vi "Open Dev Ex.vi"(7 "FuncNo":u8, 9 "DevNo":u8, 10 "busNo":u8, 11 "devId":i32) -> (2 "function return":i32, 3 "devId out":i32)   [LabVIEW 2013, in "CHR34XXX.lvlib"]
doc: "DLL BOOL __stdcall CHR34XXX_OpenDev(IN int devId); DLL BOOL __stdcall CHR34XXX_OpenDevEx(OUT int *devId,IN BYTE busNo,IN BYTE DevNo,IN BYTE FuncNo);"
uses:
  CHR34XXX.lvlib
  CHR34XXX.dll
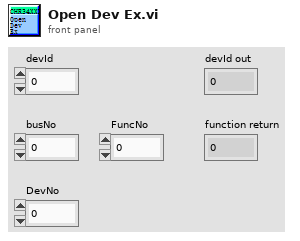
[diagram p1: front panel]
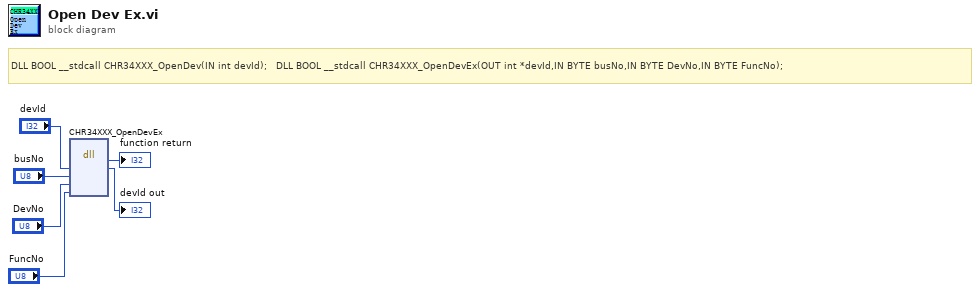
[diagram p0: block diagram]
diagram:
  # "DLL BOOL __stdcall CHR34XXX_OpenDev(IN int devId);   DLL BOOL __stdcall CHR34XXX_OpenDevEx(OUT int *devId,IN BYTE busNo,IN BYTE DevNo,IN BYTE FuncNo);"
  n1 = dll-call lib="C:/Users/dy/Desktop/CHR34XXX_lv/lv_lib/CHR34XXX.*" fn="CHR34XXX_OpenDevEx"("devId"="devId", "busNo"="busNo", "DevNo"="DevNo", "FuncNo"="FuncNo") -> (→"function return":i32, "devId"=→"devId out":i32)  [unwired: 6 in, 2 out]
